vi "RequestTags.vi"() -> (3 "Tags out":string)   [LabVIEW 2022 SP3]
uses:
  <vilib>/Utility/error.llb/Trim Whitespace One-Sided.vi
panel:
  out "Array":i32[](array[numeric])
  in  "OK Button":bool
  in  "Cancel Button":bool
  in  "Tags":i32(listbox)
  # "Double Click to Select a tag(s)"
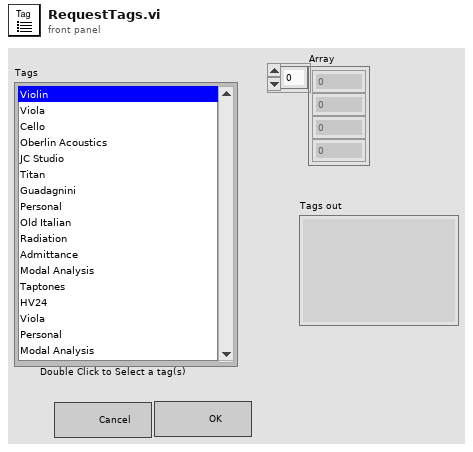
[diagram p1: front panel]
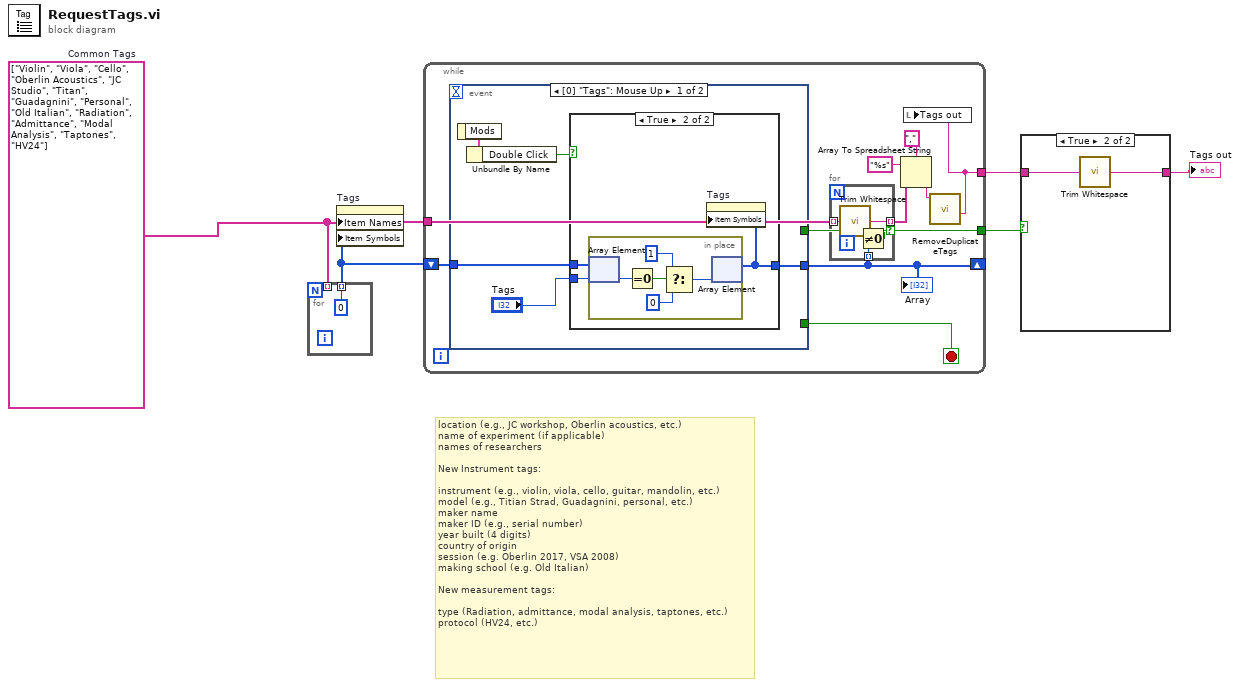
[diagram p0: block diagram]
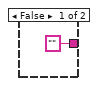
[diagram p2: hidden frame]
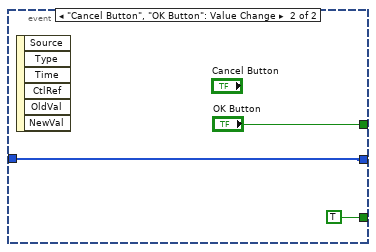
[diagram p4: hidden frame]
diagram:
  w1 = string[] ["Violin", "Viola", "Cello", "Oberlin Acoustics", "JC Studio", "Titan", "Guadagnini", "Personal", "Old Italian", "Radiation", "Admittance", "Modal Analysis", "Taptones", "HV24"]  # Common Tags
  # "location (e.g., JC workshop, Oberlin acoustics, etc.)\nname of experiment (if applicable) \nnames of researchers\n\nNew Instrument tags: \n\ninstrument (e.g., violin, viola, cello, guitar, mandolin, etc.) \nmodel (e.g., Titian Strad, Guadagnini, personal, etc.) \nmaker name\nmaker ID (e.g., serial number)\nyear built (4 digits)\ncountry of origin \nsession (e.g. Oberlin 2017, VSA 2008) \nmaking school (e.g. Old Italian) \n\nNew measurement tags: \n\ntype (Radiation, admittance, modal analysis, taptones, etc.) \nprotocol (HV24, etc.)"
  n1 = for {
    tunnel: w1 -> [_] mode=indexing
    tunnel: [0] -> w4 mode=indexing
  }
  n2 = property on="Tags" class="LstBox (strict)"("Item Names"=w1, "Item Symbols"=w4) -> ()  [unwired: 2 in, 2 out]
  n3 = while {
    tunnel: [w16] -> w5
    shift-right: [w9] -> _
    shift-left: w4 -> [w14]
    tunnel: w1 -> [w11]
    tunnel: [w7] -> w2
    stop <- w15 stop-if-true
    n4 = event shown="[0] \"Tags\": Mouse Up" {
      selector: _ -> [_ _]
      dyn-events: _ -> [_ _]
      timeout: _ -> [_ _]
      tunnel: [_ "OK Button"] -> w16
      tunnel: [_ TRUE] -> w15
      tunnel: w14 -> [w23 w35]
      tunnel: [w21 w35] -> w9
      event "Tags": Mouse Up {
        n5 = event-data() -> ("Mods"=w25:cluster{"Double Click":bool, "Menu Key":bool})  [unwired: 1 in]
        n6 = Unbundle By Name(w25) -> ("Double Click"=w24:bool)
        n7 = case shown="True" w24 {
          tunnel: w23 -> [w26 w29]
          tunnel: "Tags" -> [_ w28]
          tunnel: [w26 w27] -> w21
          frame False {
          }
          frame True {
            n8 = in-place {
              n9 = in-place-array #1(w29, w28) -> (w34:i32)
              n10 = Equal To 0?(x=w34) -> (x = 0?=w33:bool)
              n11 = Select(t=1, s=w33, f=0) -> (s? t:f=w32:i32)
              n12 = in-place-array #1(w32) -> (w27:i32[])  [unwired: 1 out]
            }
            n13 = property on="Tags" class="LstBox (strict)"("Item Symbols"=w27) -> ()  [unwired: 2 in, 2 out]
          }
        }
      }
      event "Cancel Button", "OK Button": Value Change {
        n14 = event-data() -> ()  [unwired: 1 in, 6 out]
      }
    }
    "Array" <- w9
    n15 = for {
      tunnel: w11 -> [w20] mode=indexing
      tunnel: [w17] -> w10 mode=indexing if=w18
      tunnel: w9 -> [w19] mode=indexing
      n16 = call <vilib>:"Trim Whitespace.vi"("string"=w20) -> ("trimmed string"=w17:string)  [unwired: 1 in]
      n17 = Not Equal To 0?(x=w19) -> (x != 0?=w18:bool)
    }
    n18 = Array To Spreadsheet String(delimiter (Tab)=",", array=w10, 3:"%s" ("format string")) -> (spreadsheet string=w8:string)
    n19 = call "RemoveDuplicateTags.vi"("Tags"=w8) -> ("Tag string"=w7:string)  [unwired: 9 in, 1 out]
    n20 = local write "Tags out"(w7) -> ()
  }
  n21 = case shown="True" w5 {
    tunnel: ["" ("spreadsheet string") w39] -> w3
    tunnel: w2 -> [_ w40]
    frame False {
    }
    frame True {
      n22 = call <vilib>:"Trim Whitespace.vi"("string"=w40) -> ("trimmed string"=w39:string)  [unwired: 1 in]
    }
  }
  "Tags out" <- w3
